vi "Histogram Filter.vi"() -> ()   [LabVIEW 2017]
uses:
  <vilib>/Analysis/NI_AALBase.lvlib
panel:
  in  "X Values":dbl[](array[numeric])
  out "kPk (x)":dbl[](array[numeric])
  out "k (x)":dbl[](array[numeric]) format="%0.2f"
  out "Pk(x)":i32[](array[numeric])
  out "X Scale":dbl[](array[numeric])
  out "Histogram X":T1(graph)
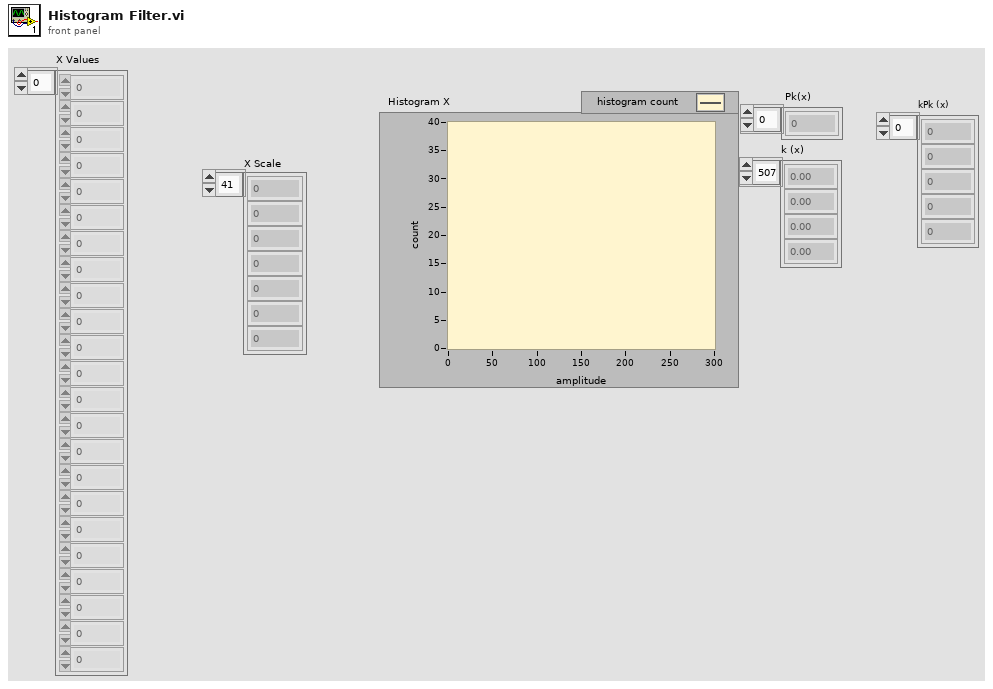
[diagram p1: front panel]
types:
  T1 = cluster{"X Values":dbl[], "Histogram: h(x)":i32[]}
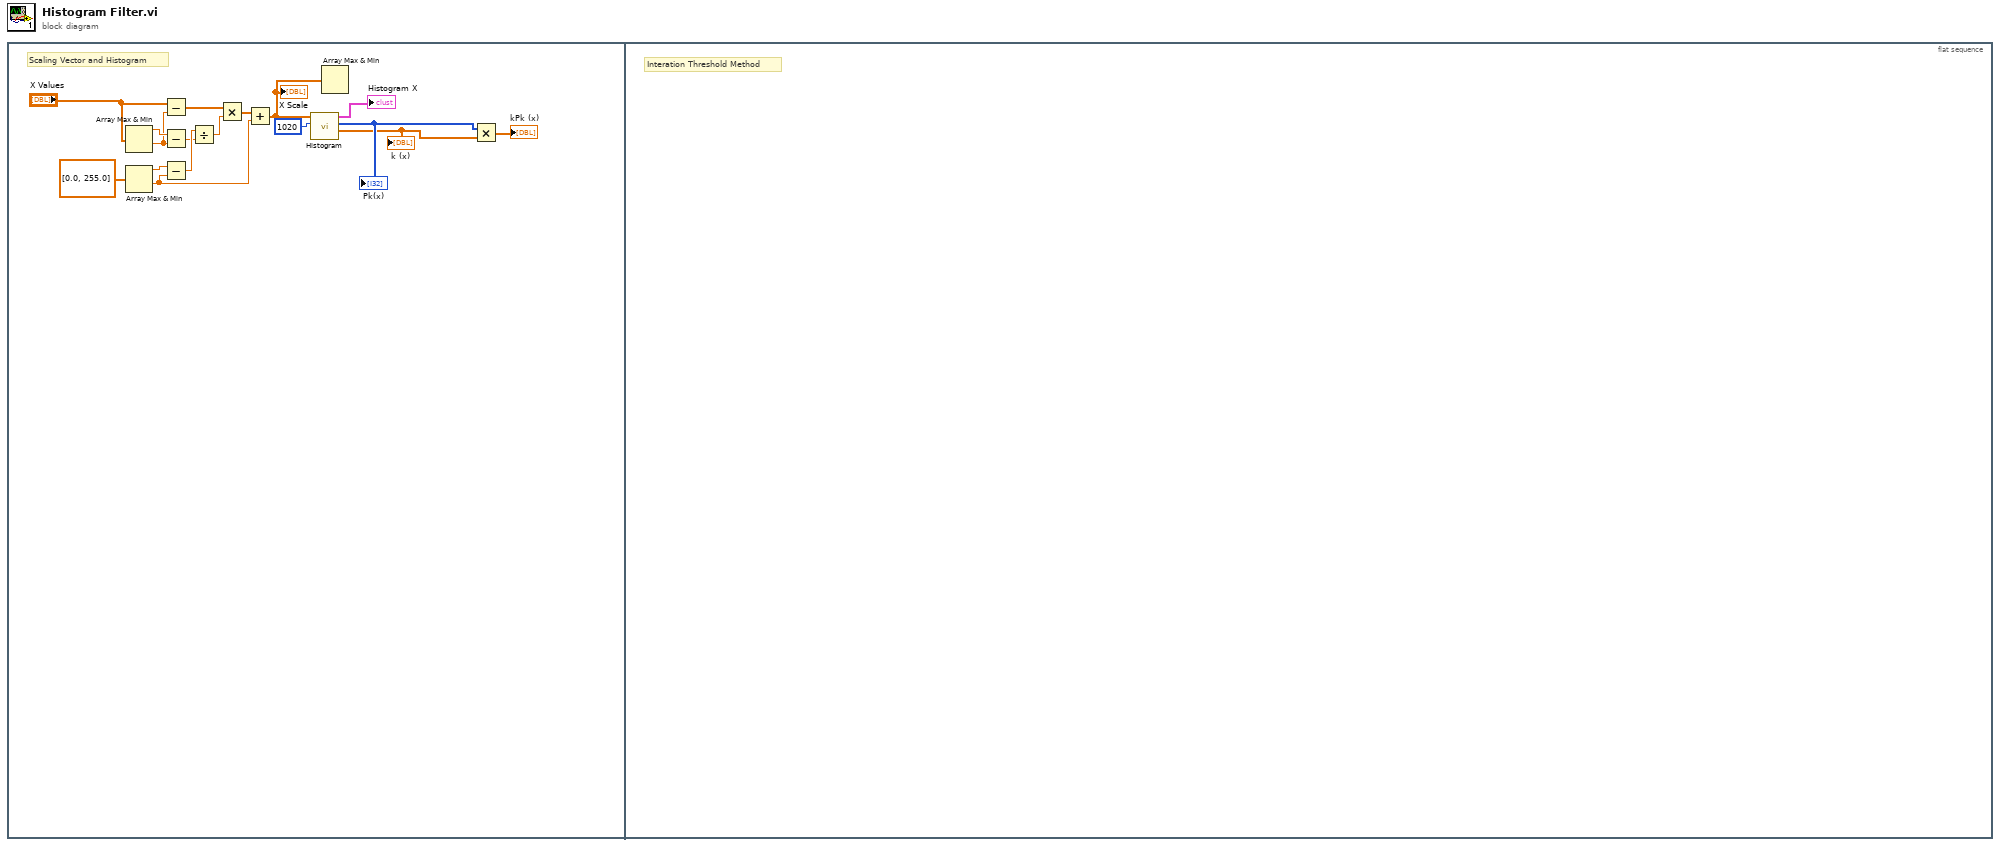
[diagram p0: block diagram]
diagram:
  n1 = flat-sequence {
    frame #0 {
      # "Scaling Vector and Histogram"
      n2 = Array Max & Min(array="X Values") -> (max value=w16:dbl, min value=w12:dbl)  [unwired: 2 out]
      n3 = Array Max & Min(array=dbl[] [0.0, 255.0]) -> (max value=w15:dbl, min value=w8:dbl)  [unwired: 2 out]
      n4 = Subtract(x="X Values", y=w12) -> (x-y=w11:dbl[])
      n5 = Subtract(x=w16, y=w12) -> (x-y=w13:dbl)
      n6 = Subtract(x=w15, y=w8) -> (x-y=w14:dbl)
      n7 = Divide(x=w14, y=w13) -> (x/y=w10:dbl)
      n8 = Multiply(x=w11, y=w10) -> (x*y=w9:dbl[])
      n9 = Add(x=w9, y=w8) -> (x+y=w2:dbl[])
      "X Scale" <- w2
      n10 = call <vilib>:"Histogram.vi"("intervals"=1020, "X"=w2) -> ("X Values"=w4:dbl[], "Histogram: h(x)"=w5:i32[], "Histogram Graph"=→"Histogram X":T1)  [unwired: 6 in, 1 out]
      "Pk(x)" <- w5
      "k (x)" <- w4
      n11 = Array Max & Min(array=w2) -> ()  [unwired: 4 out]
      n12 = Multiply(x=w5, y=w4) -> (x*y=→"kPk (x)":dbl[])
    }
    frame #1 {
      # "Interation Threshold Method"
    }
  }
